vi "AutoVision.vi"(0 "Parameters (Caliper 1)":T1(array[cluster])=[{"Feature"=0, "Points IDs"=[{"GUID"="box", "Index"=1}, {"GUID"="Tape", "Index"=1}]}] {"Feature" items=["Distance", "Mid Point", "Perpendicular Projection", "Lines Intersection", "Angle from Horizontal", "Angle from Vertical", "Angle Defined by 3 Points", "Angle Defined by 4 Points", "Bissecting Line", "Mid Line", "Center of Mass", "Area", "Line Fit", "Circle Fit", "Ellipse Fit"]}, 7 "error in":errorcluster) -> (20 "Caliper Results (Caliper 1)":sgl[][](array[numeric]) format="%.2f", 21 "Calibrated Results (Caliper 1)":sgl[][](array[numeric]) format="%.2f", 27 "error out":errorcluster)   [LabVIEW 2014]
uses:
  <vilib>/vision/driver/NI_Vision_Acquisition_Software.lvlib
  <vilib>/vision/NI_Vision_Development_Module.lvlib
panel:
  out "Image Out":T2(plugin-control)
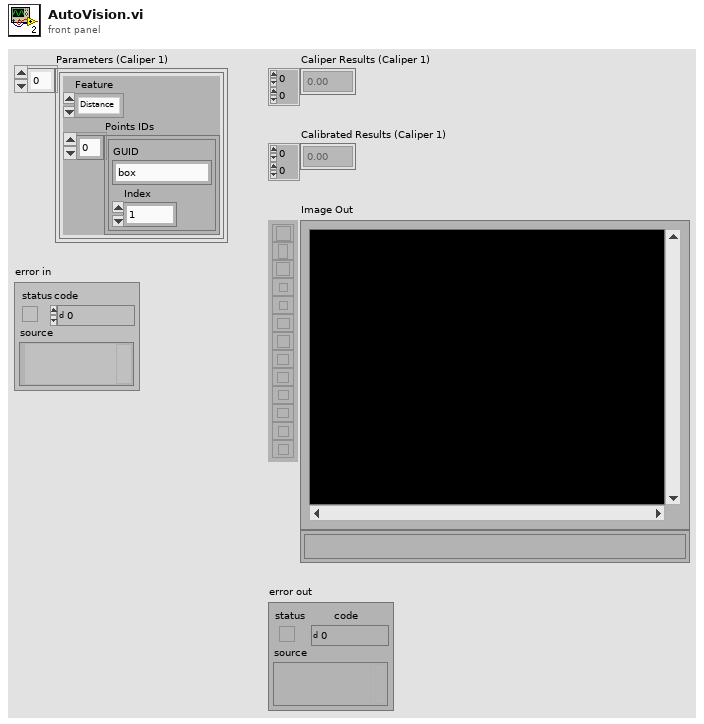
[diagram p1: front panel]
types:
  T1 = cluster{"Feature":u32, "Points IDs":cluster{"GUID":string, "Index":i32}[]}[]
  T2 = typedef "IMAQ Image.ctl" = refnum<image>
  T3 = typedef "Image Type" = u32
  T4 = cluster{"Global Rectangle":i32[], "Contours":cluster{"ID":enum32{"External", "Internal"}, "Type":u32, "Coordinates":i32[]}[]}
  T5 = typedef "IMAQdx.ctl" = refnum<k21>
  T6 = cluster{"Position":cluster{"x":sgl, "y":sgl}, "Angle":sgl, "Scale":sgl, "Score":sgl, "Bounding Box":cluster{"x":sgl, "y":sgl}[]}[]
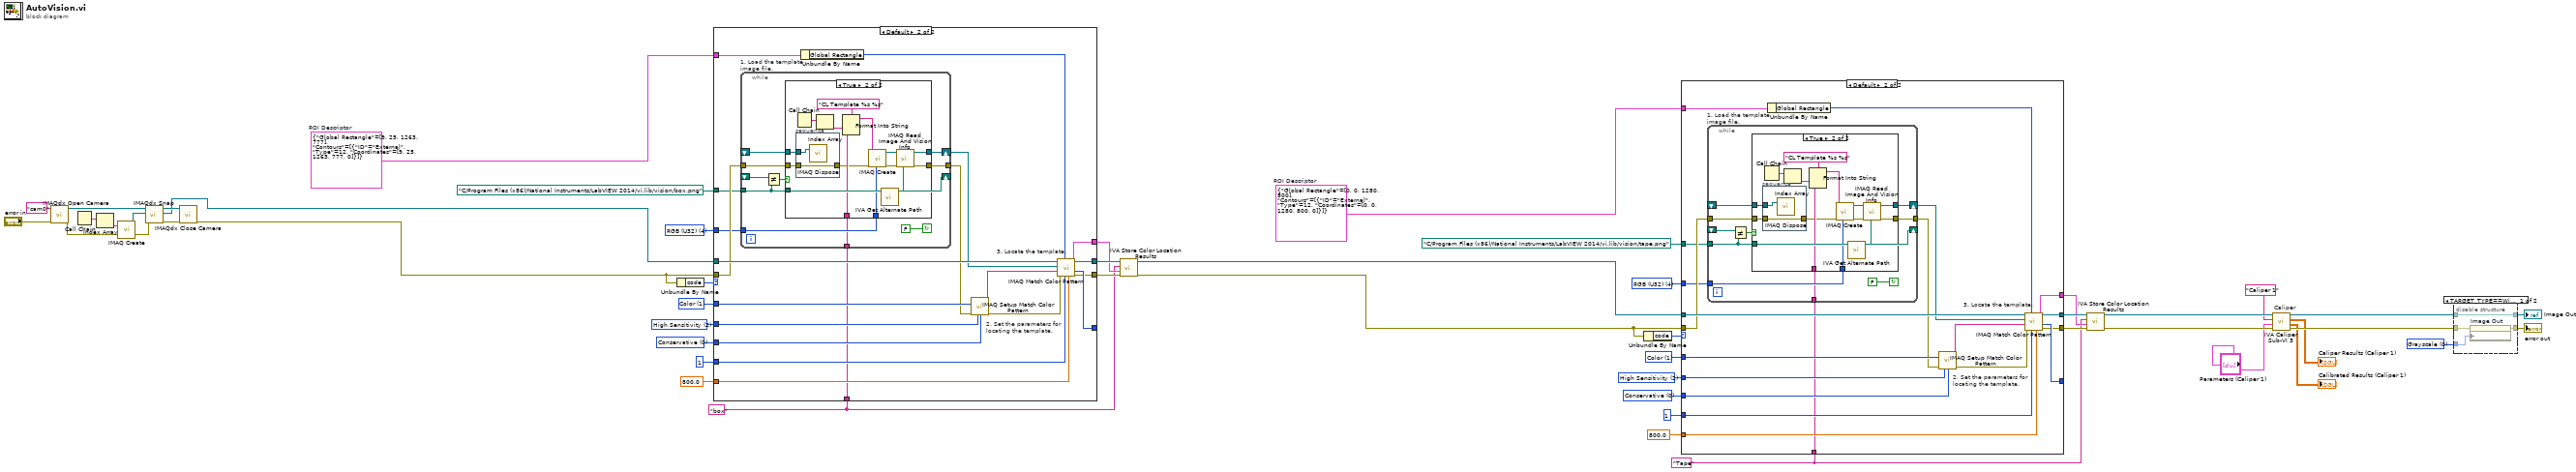
[diagram p0: block diagram]
diagram:
  w1 = u32 0 items=["Grayscale", "Binary", "Gradient", "Rainbow", "Temperature", "User Defined"] ("Palette")
  w11 = "Tape" ("Step Name")
  w19 = T3 4 items=["Grayscale (U8)", "Grayscale (I16)", "Grayscale (SGL)", "Complex (CSG)", "RGB (U32)", "HSL (U32)", "RGB (U64)"] ("Image Type")
  w21 = u32 0 items=["Conservative", "Balance", "Aggressive", "Very Aggressive"] ("Search Strategy")
  w22 = u32 2 items=["Low Sensitivity", "Medium Sensitivity", "High Sensitivity"] ("Color Sensitivity")
  w23 = u32 1 items=["Color and Shape", "Color", "Shape"] ("Match Feature Mode")
  w18 = T4 {"Global Rectangle"=[0, 0, 1280, 800], "Contours"=[{"ID"=enum."External", "Type"=12, "Coordinates"=[0, 0, 1280, 800, 0]}]}  # ROI Descriptor
  w26 = "box" ("Step Name")
  w34 = T3 4 items=["Grayscale (U8)", "Grayscale (I16)", "Grayscale (SGL)", "Complex (CSG)", "RGB (U32)", "HSL (U32)", "RGB (U64)"] ("Image Type")
  w36 = u32 0 items=["Conservative", "Balance", "Aggressive", "Very Aggressive"] ("Search Strategy")
  w37 = u32 2 items=["Low Sensitivity", "Medium Sensitivity", "High Sensitivity"] ("Color Sensitivity")
  w38 = u32 1 items=["Color and Shape", "Color", "Shape"] ("Match Feature Mode")
  w33 = T4 {"Global Rectangle"=[9, 25, 1263, 777], "Contours"=[{"ID"=enum."External", "Type"=12, "Coordinates"=[9, 25, 1263, 777, 0]}]}  # ROI Descriptor
  # "Caliper"
  n1 = call <vilib>:"IMAQdx Open Camera.vi"("error in"="error in", "Session In"="cam0" ("Interface Name")) -> ("error out"=w50:errorcluster, "Session Out"=w44:T5)  [unwired: 1 in, 7 out]
  n2 = Call Chain() -> (call chain=w42:string[])
  n3 = Index Array(array=w42) -> (element=w41:string)  [unwired: 1 in]
  n4 = call "IMAQ Create"("Image Name"=w41, "error in (no error)"=w50) -> ("New Image"=w46:T2, "error out"=w45:errorcluster)  [unwired: 2 in, 1 out]
  n5 = call <vilib>:"IMAQdx Snap.vi"("error in"=w45, "Image In"=w46, "Session In"=w44) -> ("error out"=w48:errorcluster, "Image Out"=w32:T2, "Session Out"=w49:T5)  [unwired: 6 out]
  n6 = call <vilib>:"IMAQdx Close Camera.vi"("error in"=w48, "Session In"=w49) -> ("error out"=w47:errorcluster)  [unwired: 9 out]
  n7 = Unbundle By Name(w47) -> ("code"=w31:i32)
  n8 = case shown="Default" w31 {
    tunnel: sgl 800.0 ("Minimum Match Score") -> [_ w71]
    tunnel: 1 ("Number of Matches Requested") -> [_ w70]
    tunnel: [_ w69] -> _
    tunnel: w38 -> [_ w68]
    tunnel: w37 -> [_ w67]
    tunnel: w36 -> [_ w66]
    tunnel: path "C:/Program Files (x86)/National Instruments/LabVIEW 2014/vi.lib/vision/box.png" ("File Path") -> [_ w58]
    tunnel: w34 -> [_ w57]
    tunnel: w47 -> [_ w59]
    tunnel: w33 -> [_ w63]
    tunnel: [_ w61] -> w27
    tunnel: w32 -> [w52 w60]
    tunnel: [w52 w60] -> w28
    tunnel: [_ w54] -> w29
    tunnel: w26 -> [_ w53]
    frame -1074396199, -1074396198 {
      # "Discard Coordinate System Error"
    }
    frame Default {
      # "3. Locate the template."
      # "2. Set the parameters for\nlocating the template."
      n9 = while "1. Load the template image file." {
        shift-right: [w81] -> w56
        shift-left: _ -> [w80]
        tunnel: [w78] -> w55
        tunnel: w59 -> [w77]
        tunnel: w58 -> [w72]
        tunnel: w57 -> [w76]
        tunnel: w53 -> [w75]
        shift-right: [w72] -> _
        shift-left: _ -> [w74]
        stop <- FALSE continue-if-true
        n10 = Not Equal?(x=w74, y=w72) -> (x != y?=w73:bool)
        n11 = case shown="True" w73 {
          tunnel: [w83 w96] -> w81
          tunnel: w80 -> [w83 w88]
          tunnel: [w82 w93] -> w78
          tunnel: w77 -> [w82 w87]
          tunnel: w76 -> [_ w92]
          tunnel: w75 -> [_ w89]
          tunnel: w72 -> [_ w85]
          frame False {
          }
          frame True {
            n12 = Call Chain() -> (call chain=w91:string[])
            n13 = stacked-sequence {
              tunnel: w88 -> [w100]
              tunnel: w87 -> [w99]
              tunnel: [w99] -> w86
              frame #0 {
                n14 = call "IMAQ Dispose"("Image"=w100) -> ()  [unwired: 2 in, 4 out]
              }
            }
            n15 = Index Array(array=w91) -> (element=w90:string)  [unwired: 1 in]
            n16 = Format Into String(format string="CL Template %s %s" ("Image Name"), w90, w89) -> (resulting string=w98:string)  [unwired: 2 in, 1 out]
            n17 = call "IMAQ Create"("Image Name"=w98, "Image Type"=w92, "error in (no error)"=w86) -> ("New Image"=w95:T2, "error out"=w94:errorcluster)  [unwired: 1 in, 1 out]
            n18 = call <vilib>:"IVA Get Alternate Path.vi"("Path In"=w85) -> ("Path Out"=w84:path)  [unwired: 10 out]
            n19 = call "IMAQ Read Image And Vision Info"("File Path"=w84, "error in (no error)"=w94, "Image"=w95) -> ("error out"=w93:errorcluster, "Image Out"=w96:T2)  [unwired: 1 in, 6 out]
          }
        }
      }
      n20 = Unbundle By Name(w63) -> ("Global Rectangle"=w62:i32[])
      n21 = call "IMAQ Setup Match Color Pattern"("Match Feature Mode"=w68, "error in (no error)"=w55, "Color Sensitivity"=w67, "Search Strategy"=w66) -> ("Match Color Pattern Setup Data"=w65:string, "error out"=w64:errorcluster)  [unwired: 5 in, 5 out]
      n22 = call "IMAQ Match Color Pattern"("Minimum Match Score"=w71, "Number of Matches Requested"=w70, "Optional Rectangle"=w62, "error in (no error)"=w64, "Match Color Pattern Setup Data"=w65, "Template Image"=w56, "Image"=w60) -> ("error out"=w54:errorcluster, "Number of Matches"=w69:i32, "Matches"=w61:T6)  [unwired: 2 out]
    }
  }
  n23 = call <vilib>:"IVA Store Color Location Results.vi"("error in (no error)"=w29, "Matches"=w27, "Step Name"=w26, "Image in"=w28) -> ("error out"=w30:errorcluster, "Image dup"=w17:T2)  [unwired: 6 out]
  n24 = Unbundle By Name(w30) -> ("code"=w16:i32)
  n25 = case shown="Default" w16 {
    tunnel: sgl 800.0 ("Minimum Match Score") -> [_ w120]
    tunnel: 1 ("Number of Matches Requested") -> [_ w119]
    tunnel: [_ w118] -> _
    tunnel: w23 -> [_ w117]
    tunnel: w22 -> [_ w116]
    tunnel: w21 -> [_ w115]
    tunnel: path "C:/Program Files (x86)/National Instruments/LabVIEW 2014/vi.lib/vision/tape.png" ("File Path") -> [_ w107]
    tunnel: w19 -> [_ w106]
    tunnel: w30 -> [_ w108]
    tunnel: w18 -> [_ w112]
    tunnel: [_ w110] -> w12
    tunnel: w17 -> [w101 w109]
    tunnel: [w101 w109] -> w13
    tunnel: [_ w103] -> w14
    tunnel: w11 -> [_ w102]
    frame -1074396199, -1074396198 {
      # "Discard Coordinate System Error"
    }
    frame Default {
      # "3. Locate the template."
      # "2. Set the parameters for\nlocating the template."
      n26 = while "1. Load the template image file." {
        shift-right: [w130] -> w105
        shift-left: _ -> [w129]
        tunnel: [w127] -> w104
        tunnel: w108 -> [w126]
        tunnel: w107 -> [w121]
        tunnel: w106 -> [w125]
        tunnel: w102 -> [w124]
        shift-right: [w121] -> _
        shift-left: _ -> [w123]
        stop <- FALSE continue-if-true
        n27 = Not Equal?(x=w123, y=w121) -> (x != y?=w122:bool)
        n28 = case shown="True" w122 {
          tunnel: [w132 w145] -> w130
          tunnel: w129 -> [w132 w137]
          tunnel: [w131 w142] -> w127
          tunnel: w126 -> [w131 w136]
          tunnel: w125 -> [_ w141]
          tunnel: w124 -> [_ w138]
          tunnel: w121 -> [_ w134]
          frame False {
          }
          frame True {
            n29 = Call Chain() -> (call chain=w140:string[])
            n30 = stacked-sequence {
              tunnel: w137 -> [w149]
              tunnel: w136 -> [w148]
              tunnel: [w148] -> w135
              frame #0 {
                n31 = call "IMAQ Dispose"("Image"=w149) -> ()  [unwired: 2 in, 4 out]
              }
            }
            n32 = Index Array(array=w140) -> (element=w139:string)  [unwired: 1 in]
            n33 = Format Into String(format string="CL Template %s %s" ("Image Name"), w139, w138) -> (resulting string=w147:string)  [unwired: 2 in, 1 out]
            n34 = call "IMAQ Create"("Image Name"=w147, "Image Type"=w141, "error in (no error)"=w135) -> ("New Image"=w144:T2, "error out"=w143:errorcluster)  [unwired: 1 in, 1 out]
            n35 = call <vilib>:"IVA Get Alternate Path.vi"("Path In"=w134) -> ("Path Out"=w133:path)  [unwired: 10 out]
            n36 = call "IMAQ Read Image And Vision Info"("File Path"=w133, "error in (no error)"=w143, "Image"=w144) -> ("error out"=w142:errorcluster, "Image Out"=w145:T2)  [unwired: 1 in, 6 out]
          }
        }
      }
      n37 = Unbundle By Name(w112) -> ("Global Rectangle"=w111:i32[])
      n38 = call "IMAQ Setup Match Color Pattern"("Match Feature Mode"=w117, "error in (no error)"=w104, "Color Sensitivity"=w116, "Search Strategy"=w115) -> ("Match Color Pattern Setup Data"=w114:string, "error out"=w113:errorcluster)  [unwired: 5 in, 5 out]
      n39 = call "IMAQ Match Color Pattern"("Minimum Match Score"=w120, "Number of Matches Requested"=w119, "Optional Rectangle"=w111, "error in (no error)"=w113, "Match Color Pattern Setup Data"=w114, "Template Image"=w105, "Image"=w109) -> ("error out"=w103:errorcluster, "Number of Matches"=w118:i32, "Matches"=w110:T6)  [unwired: 2 out]
    }
  }
  n40 = call <vilib>:"IVA Store Color Location Results.vi"("error in (no error)"=w14, "Matches"=w12, "Step Name"=w11, "Image in"=w13) -> ("error out"=w15:errorcluster, "Image dup"=w10:T2)  [unwired: 6 out]
  n41 = call <vilib>:"IVA Caliper Sub-VI 3.vi"("error in"=w15, "Parameters"="Parameters (Caliper 1)", "Step Name"="Caliper 1", "Image In"=w10) -> ("error out"=w9:errorcluster, "Results (Calibrated)"=→"Calibrated Results (Caliper 1)":sgl[][], "Results (Pixels)"=→"Caliper Results (Caliper 1)":sgl[][], "Image Out"=w3:T2)  [unwired: 1 in, 3 out]
  n42 = disable-structure "Conditional Disable Structure" shown="TARGET_TYPE==Windows" {
    disable-tunnel: w9 -> [w153 w154]
    disable-tunnel: [w152 w154] -> w4
    disable-tunnel: w3 -> [w151 w155]
    disable-tunnel: [w151 w155] -> w2
    disable-tunnel: w1 -> [w150 _]
    frame condition #0 {
      n43 = property on="Image Out" class="ImageControl"(error in=w153, "Palette:Palette Type"=w150) -> (error out=w152:errorcluster)  [unwired: 1 in, 1 out]
    }
    frame condition #1 (active) {
    }
  }
  "error out" <- w4
  "Image Out" <- w2
